vi "Read Driver Joystick.vi"   [LabVIEW 2020]
uses:
  <vilib>/Rock Robotics/WPI/Utilities/WPI_GetSetVariantRefNum.vi
  <vilib>/Rock Robotics/Network Tables/NT Write Numeric Array.vi
  <vilib>/Rock Robotics/Network Tables/NT Write Boolean Array.vi
  Framework/Robot Global Data.vi
types:
  T1 = enum16{"0", "1", "2", "3", "4", "5", "6", "7", "8", "9", "10", "11"}
  T2 = typedef "WPI_JoystickDevRef.ctl" = cluster{"Device":T3}
  T3 = typedef "WPI_JoystickDeviceEnum.ctl" = enum16{"USB 0", "USB 1", "USB 2", "USB 3", "USB 4", "USB 5"}
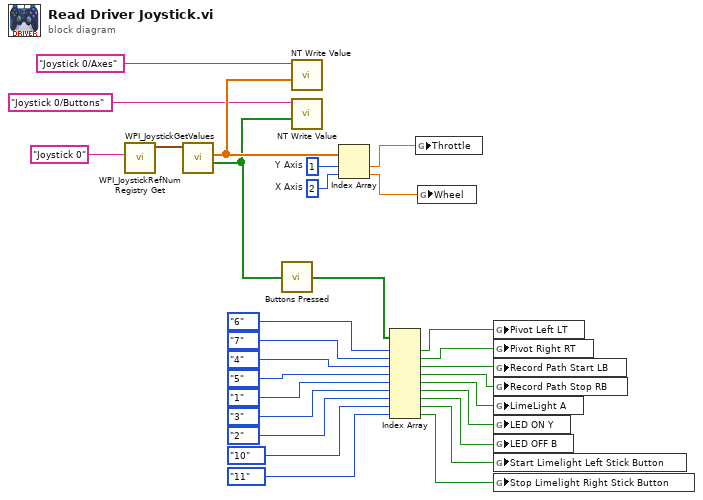
[diagram p0: block diagram]
diagram:
  w20 = 2  # X Axis
  w21 = 1  # Y Axis
  n1 = call <vilib>:"WPI_JoystickRefNum Registry Get.vi"("refnum name"="Joystick 0") -> ("JoystickDevRef"=w26:T2)  [unwired: 9 in, 1 out]
  n2 = call <vilib>:"WPI_JoystickGetValues.vi"("JoystickDevRef"=w26) -> ("Buttons"=w24:bool[], "Axes"=w29:dbl[])  [unwired: 6 in, 3 out]
  n3 = call "Buttons Pressed.vi"("Button Values"=w24) -> ("Button Presses"=w19:bool[])
  n4 = call-poly <vilib>:"NT Write Value.vi"("Numeric Array"=w29, "Name"="Joystick 0/Axes") -> ()  [unwired: 9 in, 1 out]
  n5 = call-poly <vilib>:"NT Write Value.vi"("Boolean Array"=w24, "Name"="Joystick 0/Buttons") -> ()  [unwired: 9 in, 1 out]
  n6 = Index Array(array=w29, index #1=w21, index #2=w20) -> (element #1=w23:dbl, element #2=w22:dbl)
  n7 = Index Array(array=w19, index #1=T1."6", index #2=T1."7", index #3=T1."4", index #4=T1."5", index #5=T1."1", index #6=T1."3", index #7=T1."2", index #8=T1."10", index #9=T1."11") -> (element #1=w15:bool, element #2=w16:bool, element #3=w18:bool, element #4=w17:bool, element #5=w9:bool, element #6=w8:bool, element #7=w7:bool, element #8=w2:bool, element #9=w1:bool)
  n8 = global write "Robot Global Data.vi" "Throttle"(w23) -> ()
  n9 = global write "Robot Global Data.vi" "Wheel"(w22) -> ()
  n10 = global write "Robot Global Data.vi" "Pivot Left LT"(w15) -> ()
  n11 = global write "Robot Global Data.vi" "Pivot Right RT"(w16) -> ()
  n12 = global write "Robot Global Data.vi" "Record Path Start LB"(w18) -> ()
  n13 = global write "Robot Global Data.vi" "Record Path Stop RB"(w17) -> ()
  n14 = global write "Robot Global Data.vi" "LimeLight A"(w9) -> ()
  n15 = global write "Robot Global Data.vi" "LED ON Y"(w8) -> ()
  n16 = global write "Robot Global Data.vi" "LED OFF B"(w7) -> ()
  n17 = global write "Robot Global Data.vi" "Start Limelight Left Stick Button"(w2) -> ()
  n18 = global write "Robot Global Data.vi" "Stop Limelight Right Stick Button"(w1) -> ()
